vi "DeleteExample.vi"() -> ()   [LabVIEW 2017]
uses:
  <vilib>/addons/database/Connection.llb/DB Tools Open Connec (Path).vi
  <vilib>/addons/database/NI_Database_API.lvlib
panel:
  in  "MeasurementId to delete":string
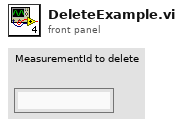
[diagram p1: front panel]
types:
  T1 = typedef "NI_Database_API.lvlib/Conn ObjectReference.ctl" = refnum<k1>
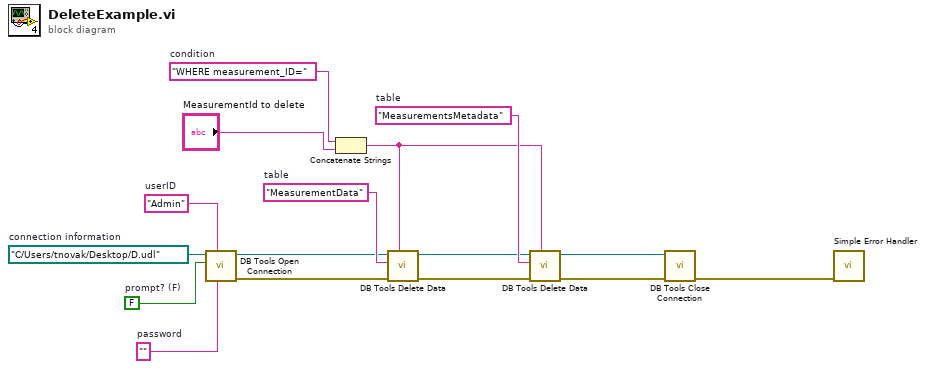
[diagram p0: block diagram]
diagram:
  w11 = path "C:/Users/tnovak/Desktop/D.udl"  # connection information
  w8 = ""  # password
  w10 = FALSE  # prompt? (F)
  w9 = "Admin"  # userID
  w14 = "MeasurementsMetadata"  # table
  w15 = "MeasurementData"  # table
  w16 = "WHERE measurement_ID="  # condition
  n1 = call-poly <vilib>:"DB Tools Open Connection.vi"("password"=w8, "userID"=w9, "prompt? (F)"=w10, "connection information"=w11) -> ("error out"=w6:errorcluster, "connection reference"=w7:T1)  [unwired: 4 in]
  n2 = Concatenate Strings(w16, "MeasurementId to delete") -> (w13:string)
  n3 = call <vilib>:"DB Tools Delete Data.vi"("condition"=w13, "error in (no error)"=w6, "table"=w15, "connection reference"=w7) -> ("error out"=w5:errorcluster, "connection reference out"=w12:T1)  [unwired: 6 in]
  n4 = call <vilib>:"DB Tools Delete Data.vi"("condition"=w13, "error in (no error)"=w5, "table"=w14, "connection reference"=w12) -> ("error out"=w2:errorcluster, "connection reference out"=w3:T1)  [unwired: 6 in]
  n5 = call <vilib>:"DB Tools Close Connection.vi"("error in (no error)"=w2, "connection reference"=w3) -> ("error out"=w4:errorcluster)  [unwired: 5 in]
  n6 = call <vilib>:"Simple Error Handler.vi"("error in (no error)"=w4) -> ()  [unwired: 4 in, 5 out]
